vi "FPGA_Read_Enc.vi"(11 "IO Cluster In":T1={"Error"={"status"=FALSE, "code"=0, "source"=""}, "Encoder Calibration Values"=[22, 216], "Update Calibration"=FALSE, "JPEG Resolutions"=3, "Raw Resolutions"=1, "Image Mode"=enum."RAW Gray Scale", "FPGA Ref"=refnum} {"JPEG Resolutions" items=["160x128"=3, "320x240"=5, "640x480"=7]; "Raw Resolutions" items=["80x60"=1, "160x120"=3, "128x128"=9, "128x96"=11]}) -> (0 "Encoder Counts":i32[](array[numeric]), 1 "Joint Coordinates (rad)":dbl[](array[numeric]), 3 "IO Cluster Out":T1={"Error"={"status"=FALSE, "code"=0, "source"=""}, "Encoder Calibration Values"=[22, 216], "Update Calibration"=FALSE, "JPEG Resolutions"=3, "Raw Resolutions"=1, "Image Mode"=enum."RAW Gray Scale", "FPGA Ref"=refnum} {"JPEG Resolutions" items=["160x128"=3, "320x240"=5, "640x480"=7]; "Raw Resolutions" items=["80x60"=1, "160x120"=3, "128x128"=9, "128x96"=11]})   [LabVIEW 2018]
uses:
  QNET MS IO Cluster.ctl
  <vilib>/Utility/error.llb/Error Cluster From Error Code.vi
  <vilib>/rvi/errors/niLvFpgaAdjustHostInterfaceError.vi
  <vilib>/rvi/interface/nirviReadWriteControl/nirviReadWriteControl.xnode
  NiFpgaLv.dll
  <vilib>/rvi/interface/Simulation/niFpgaSimulationCallBeginRW.vi
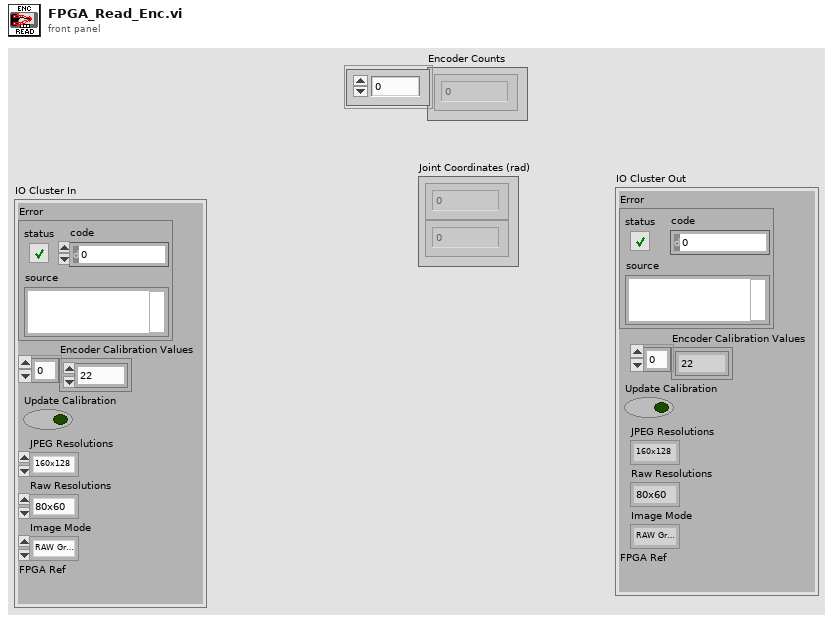
[diagram p1: front panel]
types:
  T1 = typedef "QNET MS IO Cluster.ctl" = cluster{"Error":errorcluster, "Encoder Calibration Values":i32[], "Update Calibration":bool, "JPEG Resolutions":u16, "Raw Resolutions":u16, "Image Mode":enum16{"RAW RGB", "RAW Gray Scale", "JPEG"}, "FPGA Ref":refnum<k20>}
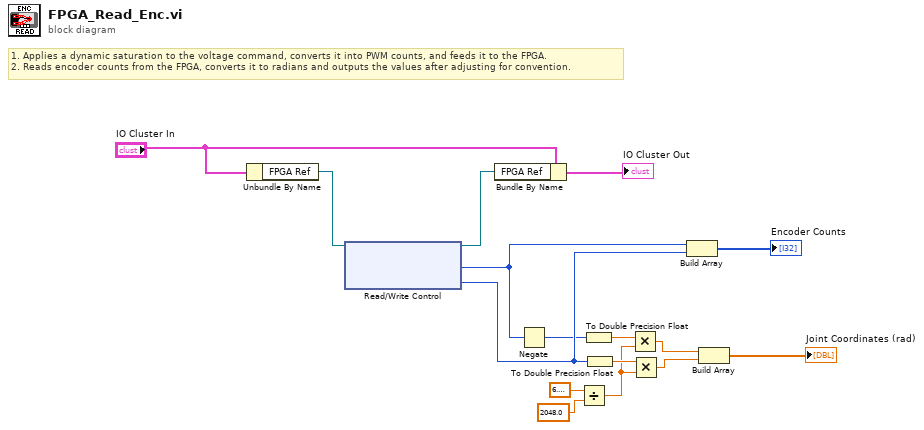
[diagram p0: block diagram]
diagram:
  # "1. Applies a dynamic saturation to the voltage command, converts it into PWM counts, and feeds it to the FPGA.\n2. Reads encoder counts from the FPGA, converts it to radians and outputs the values after adjusting for convention."
  n1 = Unbundle By Name("IO Cluster In") -> ("FPGA Ref"=w8:refnum<k20>)
  n2 = xnode ("Read/Write Control")("FPGA VI Reference In"=w8) -> ("FPGA VI Reference Out"=w7:refnum<k20>, "Encoder 0 Counter"=w1:i32, "Encoder 1 Counter"=w4:i32)  [unwired: 1 in, 1 out]
  n3 = Bundle By Name(cluster="IO Cluster In", "FPGA Ref"=w7) -> (→"IO Cluster Out":T1)
  n4 = Negate(x=w1) -> (-x=w3:i32)
  n5 = Divide(x=6.283185307179586 ("Constant 2"), y=2048.0) -> (x/y=w12:dbl)
  n6 = To Double Precision Float(number=w3) -> (double precision float=w15:dbl)
  n7 = To Double Precision Float ("To Double Precision Float 2")(number=w4) -> (double precision float=w16:dbl)
  n8 = Multiply(x=w15, y=w12) -> (x*y=w11:dbl)
  n9 = Multiply ("Multiply 2")(x=w16, y=w12) -> (x*y=w10:dbl)
  n10 = Build Array(w1, w4) -> (→"Encoder Counts":i32[])
  n11 = Build Array(w11, w10) -> (→"Joint Coordinates (rad)":dbl[])
